vi "PID Calculate P.vi"(10 "Gains":cluster{"P":dbl, "I":dbl, "D":dbl}, 11 "Error":dbl) -> ()   [LabVIEW 2014]
panel:
  out "Output":dbl
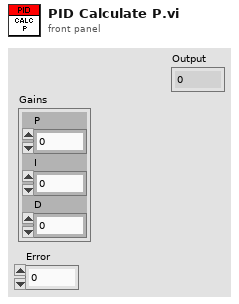
[diagram p1: front panel]
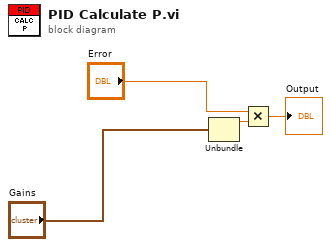
[diagram p0: block diagram]
diagram:
  n1 = Unbundle("Gains") -> ("P"=w3:dbl)  [unwired: 2 out]
  n2 = Multiply(x="Error", y=w3) -> (x*y=→"Output":dbl)
